vi "Pack AI to 24xI16 Debug.vi"(8 "Input Set4":u16[](array[numeric])=[0, 0, 0, 0, 0, 0, 0, 0] format="%.0b", 9 "Input Set3":u16[](array[numeric])=[0, 0, 0, 0, 0, 0, 0, 0] format="%016b", 10 "Input Set2":u16[](array[numeric])=[0, 0, 0, 0, 0, 0, 0, 0] format="%016b", 11 "Input Set1":u16[](array[numeric])=[0, 0, 0, 0, 0, 0, 0, 0] format="%016b") -> (0 "Output Set 3":u16[](array[numeric]) format="%016b", 1 "Output Set 2":u16[](array[numeric]) format="%016b", 2 "Output Set 1":u16[](array[numeric]) format="%016b", 3 "Output Array":u16[](array[numeric]) format="%016b")   [LabVIEW 2012]
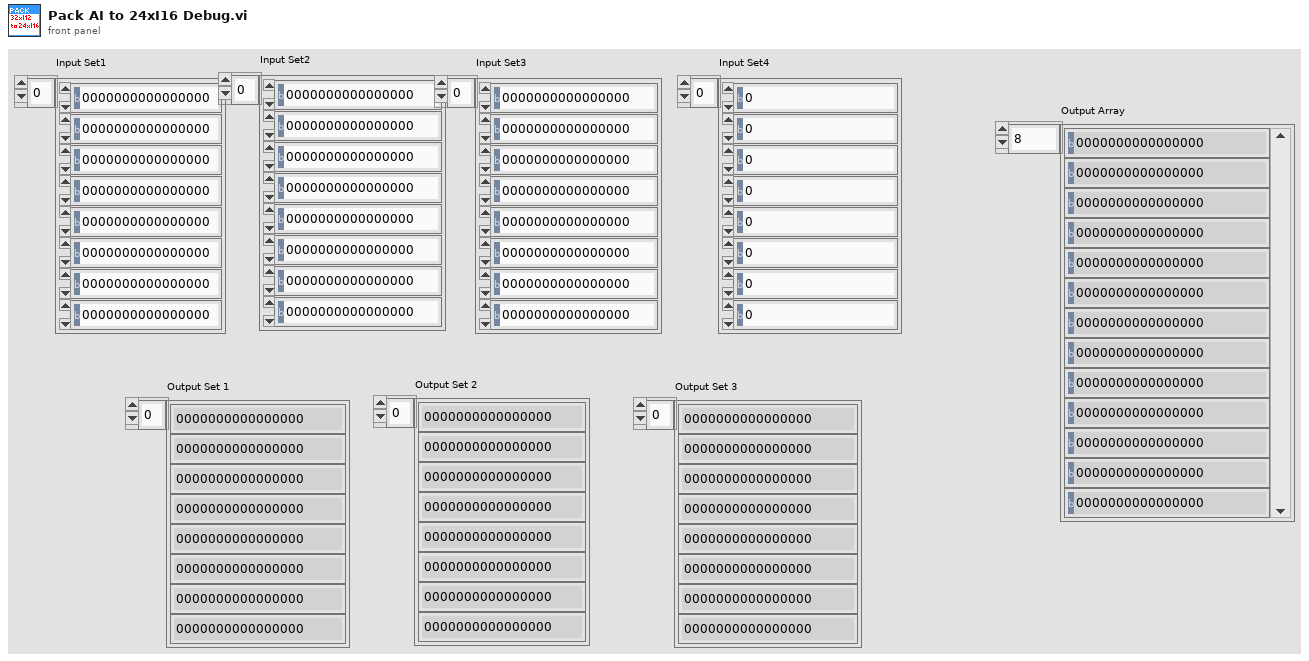
[diagram p1: front panel]
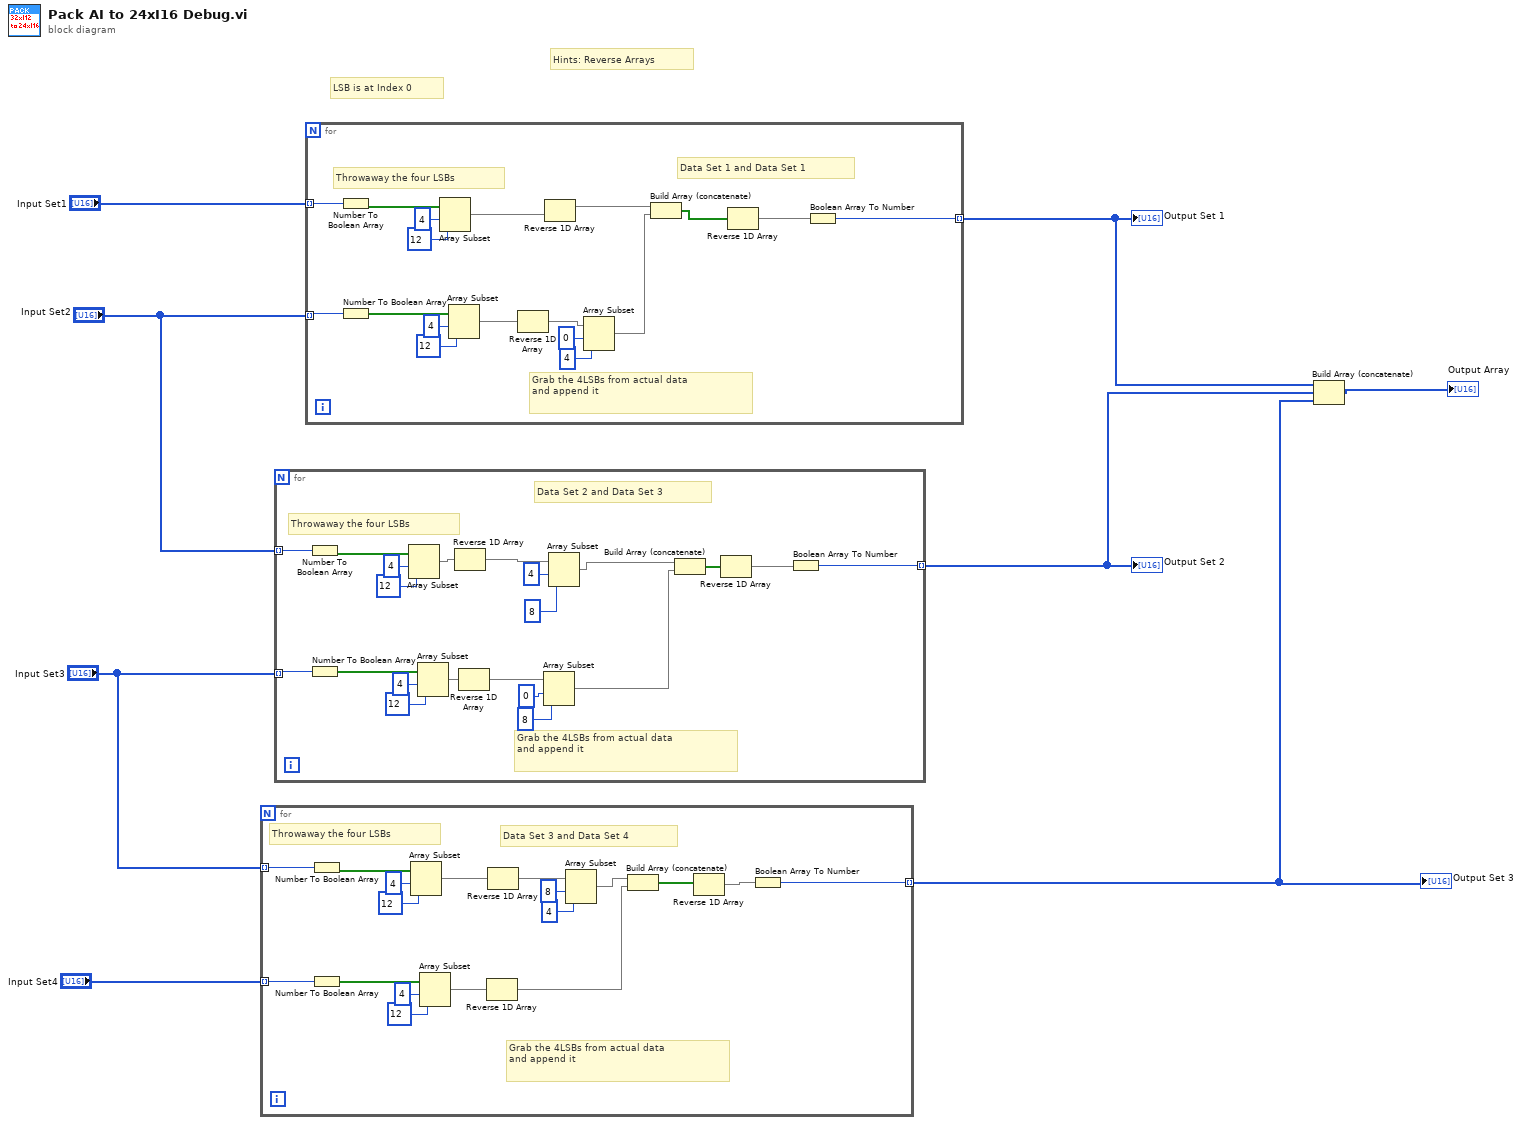
[diagram p0: block diagram]
diagram:
  # "LSB is at Index 0"
  # "Hints: Reverse Arrays"
  n1 = for {
    tunnel: "Input Set4" -> [w17] mode=indexing
    tunnel: "Input Set3" -> [w16] mode=indexing
    tunnel: [w15] -> w1 mode=indexing
    # "Data Set 3 and Data Set 4"
    # "Grab the 4LSBs from actual data \nand append it"
    # "Throwaway the four LSBs"
    n2 = Number To Boolean Array(number=w16) -> (Boolean array=w18:bool[])
    n3 = Number To Boolean Array(number=w17) -> (Boolean array=w23:bool[])
    n4 = Array Subset(array=w18, index=4, length=12 ("index")) -> (w26:bool[])
    n5 = Array Subset(array=w23, index=4, length=12 ("index")) -> (w12:bool[])
    n6 = Reverse 1D Array(array=w12) -> (reversed array=w9:bool[])
    n7 = Reverse 1D Array(array=w26) -> (reversed array=w11:bool[])
    n8 = Array Subset(array=w11, index=8, length=4 ("index")) -> (w14:bool[])
    n9 = Build Array (concatenate)(w14, w9) -> (w13:bool[])
    n10 = Reverse 1D Array(array=w13) -> (reversed array=w10:bool[])
    n11 = Boolean Array To Number(Boolean array=w10) -> (number=w15:u16)
  }
  "Output Set 3" <- w1
  n12 = for {
    tunnel: "Input Set2" -> [w47] mode=indexing
    tunnel: "Input Set3" -> [w46] mode=indexing
    tunnel: [w36] -> w3 mode=indexing
    # "Data Set 2 and Data Set 3"
    # "Grab the 4LSBs from actual data \nand append it"
    # "Throwaway the four LSBs"
    n13 = Number To Boolean Array(number=w47) -> (Boolean array=w45:bool[])
    n14 = Number To Boolean Array(number=w46) -> (Boolean array=w40:bool[])
    n15 = Array Subset(array=w45, index=4, length=12 ("index")) -> (w33:bool[])
    n16 = Array Subset(array=w40, index=4, length=12 ("index")) -> (w30:bool[])
    n17 = Reverse 1D Array(array=w33) -> (reversed array=w29:bool[])
    n18 = Reverse 1D Array(array=w30) -> (reversed array=w28:bool[])
    n19 = Array Subset(array=w28, index=0, length=8 ("index")) -> (w37:bool[])
    n20 = Array Subset(array=w29, index=4, length=8 ("index")) -> (w31:bool[])
    n21 = Build Array (concatenate)(w31, w37) -> (w32:bool[])
    n22 = Reverse 1D Array(array=w32) -> (reversed array=w27:bool[])
    n23 = Boolean Array To Number(Boolean array=w27) -> (number=w36:u16)
  }
  "Output Set 2" <- w3
  n24 = for {
    tunnel: "Input Set1" -> [w65] mode=indexing
    tunnel: "Input Set2" -> [w64] mode=indexing
    tunnel: [w52] -> w4 mode=indexing
    # "Data Set 1 and Data Set 1"
    # "Grab the 4LSBs from actual data \nand append it"
    # "Throwaway the four LSBs"
    n25 = Number To Boolean Array(number=w65) -> (Boolean array=w63:bool[])
    n26 = Number To Boolean Array(number=w64) -> (Boolean array=w58:bool[])
    n27 = Array Subset(array=w63, index=4, length=12 ("index")) -> (w55:bool[])
    n28 = Array Subset(array=w58, index=4, length=12 ("index")) -> (w51:bool[])
    n29 = Reverse 1D Array(array=w51) -> (reversed array=w49:bool[])
    n30 = Reverse 1D Array(array=w55) -> (reversed array=w50:bool[])
    n31 = Array Subset(array=w49, index=0, length=4 ("index")) -> (w54:bool[])
    n32 = Build Array (concatenate)(w50, w54) -> (w53:bool[])
    n33 = Reverse 1D Array(array=w53) -> (reversed array=w48:bool[])
    n34 = Boolean Array To Number(Boolean array=w48) -> (number=w52:u16)
  }
  "Output Set 1" <- w4
  n35 = Build Array (concatenate)(w4, w3, w1) -> (→"Output Array":u16[])
